vi "Разбор строки.vi"() -> ()   [LabVIEW 2017]
panel:
  out "Выходная подстрока":string
  out "Число":dbl
  in  "Входная строка":string
  in  "Длинна подстроки":i32
  in  "Смещение числа":i32
  in  "Смещение подстроки":i32
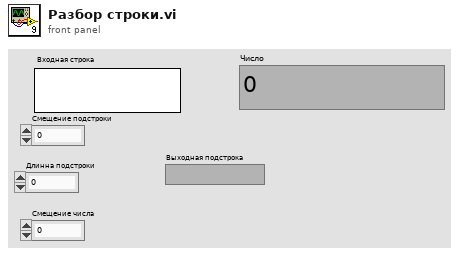
[diagram p1: front panel]
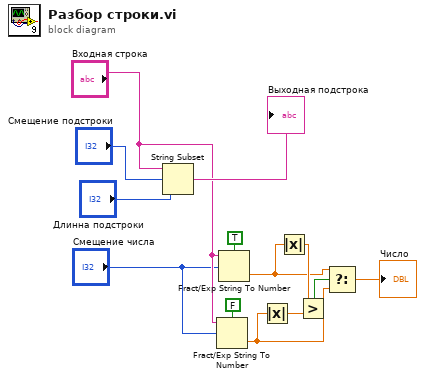
[diagram p0: block diagram]
diagram:
  n1 = String Subset(string="Входная строка", offset (0)="Смещение подстроки", length (rest)="Длинна подстроки") -> (substring=→"Выходная подстрока":string)
  n2 = Fract/Exp String To Number(use system decimal point (T)=FALSE, string="Входная строка", offset="Смещение числа") -> (number=w1:dbl)  [unwired: 1 in, 1 out]
  n3 = Fract/Exp String To Number(use system decimal point (T)=TRUE, string="Входная строка", offset="Смещение числа") -> (number=w2:dbl)  [unwired: 1 in, 1 out]
  n4 = Absolute Value(x=w1) -> (abs(x)=w4:dbl)
  n5 = Absolute Value(x=w2) -> (abs(x)=w3:dbl)
  n6 = Greater?(x=w3, y=w4) -> (0:w5:bool)
  n7 = Select(t=w2, s=w5, f=w1) -> (s? t:f=→"Число":dbl)
